vi "Turbo Pump Controller.vi"() -> ()   [LabVIEW 2012]
uses:
  Type/_Pump Parameter.ctl
panel:
  in  "Send":bool
  out "Data":string
  out "Raw Reply":string
  out "Telegram":string
  in  "Input Value":i32
  in  "Pump Command":T1
  # "For RS485 serial chanel communication with Pfeiffer turbo pump"
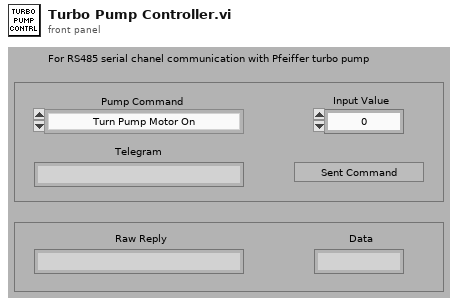
[diagram p1: front panel]
types:
  T1 = typedef "_Pump Parameter.ctl" = enum16{"Turn Pump Motor On", "Turn Pump Motor Off", "Read Pump Oil Deficiency", "Read Rotation Switch Point Attained", "Read Ele. Drive Over Temperature", "Read Pump Over Temperature", "Read Set Rotation Speed Attained", "Read Turbopump Accelerates", "Read Actual Rotation Speed in Hz", "Read Motor Current in A", "Read Operating Hours in h", "Read Motor Voltage in V", "Read Motor Power in W", "Set Rotation Speed Switchpoint in %", "Clear Error", "Read Error Code", "Read Bearing Temperature", "Read Hardware Version", "Read Firmware Version", "Read Operating Hours (Drive)", "Read Rotational Speed (rpm)", "Read Power Stage Temperature", "Read Electronics Temperature", "Read Upper Pump Temperature", "Read Motor Temperature", "Read Error Code History, 1", "Read Error Code History, 2", "Read Error Code History, 3", "Read Error Code History, 4", "Read Error Code History, 5", "Read Error Code History, 6", "Read Error Code History, 7", "Read Error Code History, 8", "Read Error Code History, 9", "Read Error Code History, 10"}
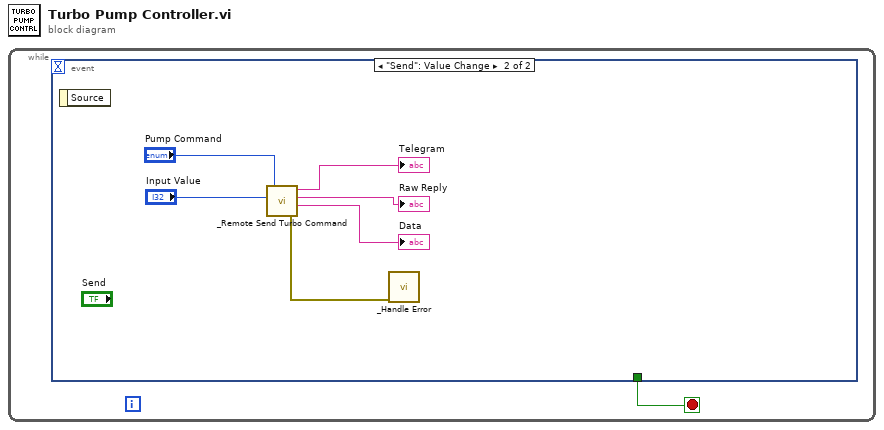
[diagram p0: block diagram]
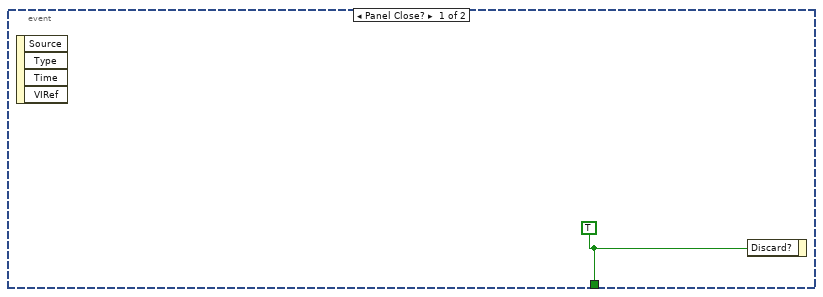
[diagram p2: hidden frame]
diagram:
  n1 = while {
    stop <- w1 stop-if-true
    n2 = event shown="[1] \"Send\": Value Change" {
      selector: _ -> [_ _]
      dyn-events: _ -> [_ _]
      timeout: _ -> [_ _]
      tunnel: [w2 _] -> w1
      event Panel Close? {
        w2 = TRUE
        n3 = event-data() -> ()  [unwired: 5 out]
        n4 = event-data("Discard?"=w2) -> ()  [unwired: 1 in, 1 out]
      }
      event "Send": Value Change {
        n5 = event-data() -> ()  [unwired: 2 out]
        n6 = call "_Remote Send Turbo Command.vi"("Input Value"="Input Value", "Pump Command"="Pump Command") -> ("error out"=w3:errorcluster, "Data"=→"Data":string, "Raw Reply"=→"Raw Reply":string, "Telegram"=→"Telegram":string)  [unwired: 1 in, 1 out]
        n7 = call "_Handle Error.vi"("error in (no error)"=w3) -> ()  [unwired: 2 in, 5 out]
      }
    }
  }
